vi "Create Plot Object.vi"(6 "Control Ref Queue":T1, 7 "Actual Transform In":T2, 8 "error in (no error)":errorcluster, 9 "Multiplot Representation In":T4, 10 "3D Comet.lvclass in":refnum<class "3D Comet.lvclass">, 11 "Plot Object In":refnum<vi>) -> (0 "error out":errorcluster, 1 "Multiplot Representation Out":T4, 2 "3D Comet.lvclass out":refnum<class "3D Comet.lvclass">, 3 "Plot Object Out":refnum<vi>, 5 "Actual Transform Out":T2)   [LabVIEW 2017, in "3D Comet.lvclass"]
uses:
  <vilib>/Math Plots/3D Math Plots/3D Comet/3D Comet/3D Comet.lvclass
  <vilib>/Math Plots/3D Math Plots/3D Plot/3D Plot/Typedef/Multiplot Representation.ctl
  <vilib>/Math Plots/3D Math Plots/3D Plot/3D Plot/Typedef/Plot Representation.ctl
  <vilib>/Math Plots/3D Math Plots/3D Plot/3D Plot/Typedef/Range Clusters.ctl
  <vilib>/Math Plots/3D Math Plots/3D Plot/3D Plot/Typedef/Mesh Data.ctl
  <vilib>/Math Plots/3D Math Plots/3D Plot/3D Plot/Typedef/Actual Transform.ctl
  <vilib>/Math Plots/3D Math Plots/3D Plot/Action String/3DMathPlot Ctrl Act Queue.ctl
  <vilib>/Math Plots/3D Math Plots/3D Plot/Action String/3DMathPlot Ctrl Act Cluster.ctl
  <vilib>/Math Plots/3D Math Plots/3D Plot/Action String/3DMathPlot State Class.ctl
  <vilib>/Math Plots/3D Math Plots/3D Comet/3D Comet/3D Comet.lvclass/3D Comet.ctl
  <vilib>/Math Plots/3D Math Plots/3D Plot/3D Plot/3D Plot.lvclass
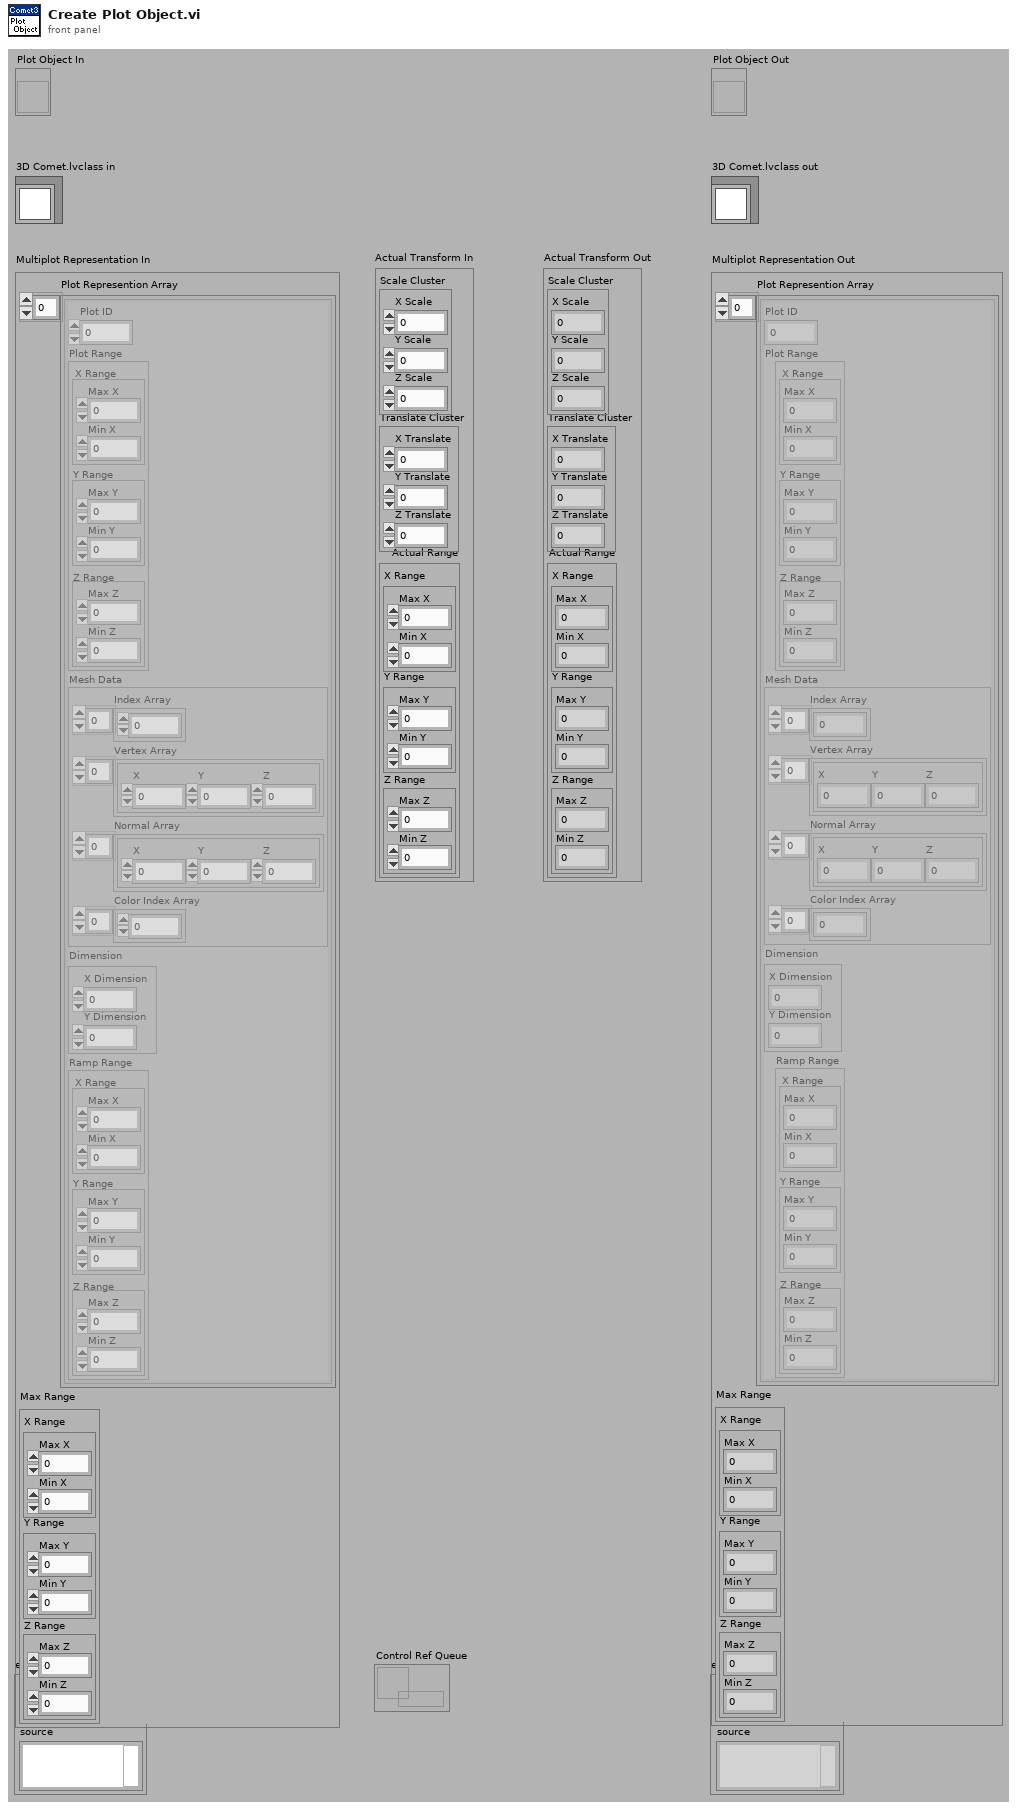
[diagram p1: front panel]
types:
  T1 = typedef "3DMathPlot Ctrl Act Queue.ctl" = refnum<queue>
  T2 = typedef "3D Plot.lvclass/Actual Transform.ctl" = cluster{"Scale Cluster":cluster{"X Scale":sgl, "Y Scale":sgl, "Z Scale":sgl}, "Translate Cluster":cluster{"X Translate":sgl, "Y Translate":sgl, "Z Translate":sgl}, "Actual Range":T3}
  T3 = typedef "3D Plot.lvclass/Range Clusters.ctl" = cluster{"X Range":cluster{"Max X":sgl, "Min X":sgl}, "Y Range":cluster{"Max Y":sgl, "Min Y":sgl}, "Z Range":cluster{"Max Z":sgl, "Min Z":sgl}}
  T4 = typedef "3D Plot.lvclass/Multiplot Representation.ctl" = cluster{"Plot Represention Array":T5[], "Max Range":T3}
  T5 = typedef "3D Plot.lvclass/Plot Representation.ctl" = cluster{"Plot ID":i32, "Plot Range":T3, "Mesh Data":T6, "Dimension":cluster{"X Dimension":i32, "Y Dimension":i32}, "Ramp Range":T3}
  T6 = typedef "3D Plot.lvclass/Mesh Data.ctl" = cluster{"Index Array":u32[], "Vertex Array":cluster{"X":sgl, "Y":sgl, "Z":sgl}[], "Normal Array":cluster{"X":sgl, "Y":sgl, "Z":sgl}[], "Color Index Array":i32[]}
  T7 = typedef "3D Comet.lvclass/3D Comet Property Array.ctl" = T8[]
  T8 = typedef "3D Comet.lvclass/3D Comet Property.ctl" = cluster{"General Property":cluster{"Plot Name":string, "Coordinate System":enum16{"Cartesian", "Cylindrical", "Spherical"}, "Opacity":sgl}, "Projection Property":cluster{"Draw XY":bool, "Draw YZ":bool, "Draw XZ":bool}, "Plot Property":cluster{"Sprite Type":T9, "Point Size":sgl, "Point Color":u32, "Line Style":T10, "Line Width":sgl, "Line Color":u32, "Antialiasing":bool}, "Comet Property":cluster{"Body length":sgl}}
  T9 = typedef "3D Plot.lvclass/Sprite Type.ctl" = enum16{"None", "Empty Square", "Solid Square", "Empty Diamond", "Solid Diamond", "Empty Circle", "Solid Circle", "Asterisk", "Bold X", "Wireframe Sphere", "Solid Sphere", "Wireframe Cube", "Solid Cube"}
  T10 = typedef "3D Plot.lvclass/Line Type.ctl" = enum16{"None", "Solid", "Dash", "Dot", "Dash Dot"}
  T11 = typedef "3DMathPlot Ctrl Act Cluster.ctl" = cluster{"3D Picture Control":refnum<vi>, "Render Window Refnum":refnum<vi>, "XY Graph":refnum<vi>, "Intensity Graph":refnum<vi>, "Color Legend Palette":refnum<vi>, "Projection Palette":refnum<vi>, "XControl  Ref":refnum<vi>, "Facade Ref":refnum<vi>, "Export Image Ref":refnum<vi>, "Clear Data Flag":bool, "Display State Change Class":T12}
  T12 = typedef "3DMathPlot State Class.ctl" = enum16{"Update All Objects (Undo)", "Update Light Object Only", "Update Axis Object Only", "Update Plot Object Only", "Update Cursor Object Only", "Update Axis Plot Cursor Objects", "No Update"}
  T13 = enum16{"Points", "Lines", "Line Strip", "Line Loop", "Triangles", "Triangle Strip", "Triangle Fan", "Quads", "Quad Strip", "Polygon"}
  T14 = cluster{"Draw XY":bool, "Draw YZ":bool, "Draw XZ":bool}
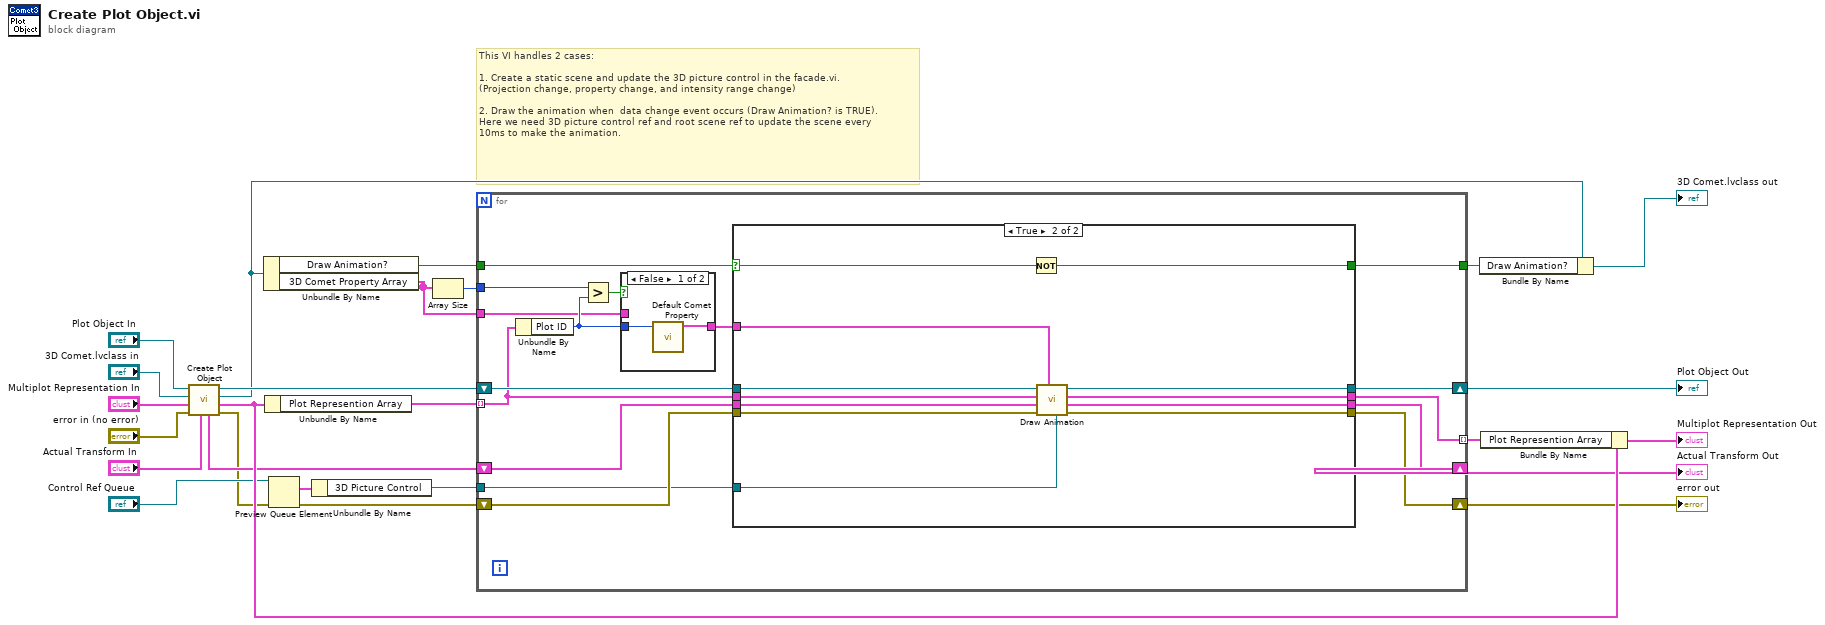
[diagram p0: block diagram]
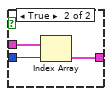
[diagram p2: hidden frame]
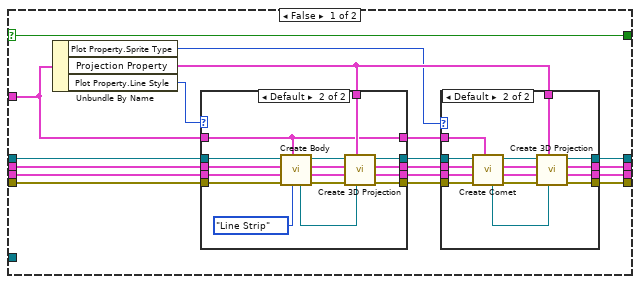
[diagram p3: hidden frame]
diagram:
  # "This VI handles 2 cases:\n\n1. Create a static scene and update the 3D picture control in the facade.vi.\n(Projection change, property change, and intensity range change)\n\n2. Draw the animation when  data change event occurs (Draw Animation? is TRUE). \nHere we need 3D picture control ref and root scene ref to update the scene every\n10ms to make the animation."
  n1 = call-parent "Create Plot Object.vi"("Actual Transform In"="Actual Transform In", "error in (no error)"="error in (no error)", "Multiplot Representation In"="Multiplot Representation In", "3D Plot.lvclass in"="3D Comet.lvclass in", "Plot Object In"="Plot Object In") -> ("error out"=w4:errorcluster, "Multiplot Representation Out"=w19:T4, "3D Plot.lvclass out"=w3:refnum<class "3D Comet.lvclass">, "Plot Object Out"=w6:refnum<vi>, "Actual Transform Out"=w11:T2)  [unwired: 2 in]
  n2 = Unbundle By Name(w3) -> ("Draw Animation?"=w13:bool, "3D Comet Property Array"=w2:T7)
  n3 = Unbundle By Name(w19) -> ("Plot Represention Array"=w21:T5[])
  n4 = Preview Queue Element(queue="Control Ref Queue", error in (no error)=w4) -> (element=w9:T11, error out=w7:errorcluster)  [unwired: 3 out]
  n5 = Unbundle By Name(w9) -> ("3D Picture Control"=w8:refnum<vi>)
  n6 = Array Size(array=w2) -> (size(s)=w1:i32)
  n7 = for {
    shift-right: [w39] -> w16
    shift-left: w7 -> [w35]
    shift-right: [w41] -> w5
    shift-left: w6 -> [w38]
    shift-right: [w40] -> w15
    shift-left: w11 -> [w36]
    tunnel: w21 -> [w37] mode=indexing
    tunnel: w2 -> [w28]
    tunnel: [w34] -> w20 mode=indexing
    tunnel: w13 -> [w31]
    tunnel: w8 -> [w33]
    tunnel: [w32] -> w12
    tunnel: w1 -> [w26]
    n8 = Unbundle By Name(w37) -> ("Plot ID"=w29:i32)
    n9 = Greater?(x=w26, y=w29) -> (0:w30:bool)
    n10 = case shown="False" w30 {
      tunnel: w28 -> [_ w46]
      tunnel: [w42 w45] -> w27
      tunnel: w29 -> [w43 w44]
      frame False {
        n11 = call <vilib>:"Default Comet Property.vi"("Plot ID"=w43) -> ("Default Property"=w42:T8)  [unwired: 10 out]
      }
      frame True {
        n12 = Index Array(array=w46, index=w44) -> (element=w45:T8)
      }
    }
    n13 = case shown="True" w31 {
      selector: w31 -> [w52 w105]
      tunnel: [w64 w109] -> w41
      tunnel: [w63 w107] -> w40
      tunnel: [w62 w106] -> w39
      tunnel: w38 -> [w61 w114]
      tunnel: w37 -> [w60 w113]
      tunnel: w36 -> [w59 w112]
      tunnel: w35 -> [w58 w111]
      tunnel: [w56 w108] -> w34
      tunnel: w27 -> [w50 w110]
      tunnel: w33 -> [_ w103]
      tunnel: [w52 w104] -> w32
      frame False {
        n14 = Unbundle By Name(w50) -> ("Plot Property.Sprite Type"=w48:T9, "Projection Property"=w51:T14, "Plot Property.Line Style"=w49:T10)
        n15 = case shown="Default" w49 {
          tunnel: w61 -> [w87 w102]
          tunnel: w60 -> [w86 w101]
          tunnel: w59 -> [w85 w100]
          tunnel: w58 -> [w84 w99]
          tunnel: [w86 w98] -> w57
          tunnel: [w87 w93] -> w55
          tunnel: [w85 w92] -> w54
          tunnel: [w84 w91] -> w53
          tunnel: w51 -> [_ w90]
          tunnel: w50 -> [w83 w88]
          tunnel: [w83 w88] -> w47
          frame "None" {
          }
          frame Default {
            n16 = call <vilib>:"Create Body.vi"("Draw Mode"=T13."Line Strip", "3D Comet Property"=w88, "error in (no error)"=w99, "Actual Transform In"=w100, "Plot Representation In"=w101, "Plot Object In"=w102) -> ("error out"=w95:errorcluster, "Actual Transform Out"=w96:T2, "Plot Representation Out"=w98:T5, "Plot Object Out"=w97:refnum<vi>, "Track Object Out"=w94:refnum<vi>)  [unwired: 1 in]
            n17 = call <vilib>:"Create 3D Projection.vi"("Sub Object In"=w94, "Projection Property"=w90, "error in (no error)"=w95, "Actual Transform In"=w96, "Plot Object In"=w97) -> ("error out"=w91:errorcluster, "Actual Transform Out"=w92:T2, "Plot Object Out"=w93:refnum<vi>)  [unwired: 1 in, 3 out]
          }
        }
        n18 = case shown="Default" w48 {
          tunnel: [w65 w82] -> w64
          tunnel: [w67 w81] -> w63
          tunnel: [w68 w80] -> w62
          tunnel: w57 -> [w66 w79]
          tunnel: [w66 w78] -> w56
          tunnel: w55 -> [w65 w77]
          tunnel: w54 -> [w67 w76]
          tunnel: w53 -> [w68 w75]
          tunnel: w51 -> [_ w70]
          tunnel: w47 -> [_ w69]
          frame "None" {
          }
          frame Default {
            n19 = call <vilib>:"Create Comet.vi"("3D Comet Property"=w69, "error in (no error)"=w75, "Actual Transform In"=w76, "Plot Representation In"=w79, "Plot Object In"=w77) -> ("error out"=w74:errorcluster, "Actual Transform Out"=w73:T2, "Plot Representation Out"=w78:T5, "Plot Object Out"=w72:refnum<vi>, "Body Object Out"=w71:refnum<vi>)  [unwired: 1 in, 1 out]
            n20 = call <vilib>:"Create 3D Projection.vi"("Sub Object In"=w71, "Projection Property"=w70, "error in (no error)"=w74, "Actual Transform In"=w73, "Plot Object In"=w72) -> ("error out"=w80:errorcluster, "Actual Transform Out"=w81:T2, "Plot Object Out"=w82:refnum<vi>)  [unwired: 1 in, 3 out]
          }
        }
      }
      frame True {
        n21 = Not(x=w105) -> (.not. x?=w104:bool)
        n22 = call <vilib>:"Draw Animation.vi"("3D Scene Ref"=w103, "3D Comet Property"=w110, "error in (no error)"=w111, "Actual Transform In"=w112, "Plot Representation In"=w113, "Plot Object In"=w114) -> ("error out"=w106:errorcluster, "Actual Transform Out"=w107:T2, "Plot Representation Out"=w108:T5, "Plot Object Out"=w109:refnum<vi>)  [unwired: 2 out]
      }
    }
  }
  "error out" <- w16
  "Plot Object Out" <- w5
  "Actual Transform Out" <- w15
  n23 = Bundle By Name(cluster=w3, "Draw Animation?"=w12) -> (→"3D Comet.lvclass out":refnum<class "3D Comet.lvclass">)
  n24 = Bundle By Name(cluster=w19, "Plot Represention Array"=w20) -> (→"Multiplot Representation Out":T4)
